vi "FromRepo.vi"(8 "error in":errorcluster, 9 "from repo cluster":T2, 10 "repository in":refnum<class "NISE_CEF_Repository.lvclass">, 11 "node in":refnum<class "VI modification collection.lvclass">) -> (0 "error out":errorcluster, 2 "repository out":refnum<class "NISE_CEF_Repository.lvclass">, 3 "node":T1)   [LabVIEW 2013, in "VI modification collection.lvclass"]
doc: "Grabs information from the Repo and stores it in the nodes."
uses:
  VI modification collection.lvclass
  <vilib>/CEF_TreeControl/Repository/NISE_CEF_Repository.lvclass
  <vilib>/CEF_TreeControl/Node/FromRepoCluster.ctl
  <vilib>/CEF_TreeControl/Node/NodeRef.ctl
  <vilib>/CEF_TreeControl/Node/NISE_CEF_Node.lvclass
  Modifier UI/modification container/modification container.lvclass
  Modifier UI/modification container/modification container.lvclass/modification container.ctl
  VI modification.lvclass
  Modifier UI/modification container/Read mods.vi
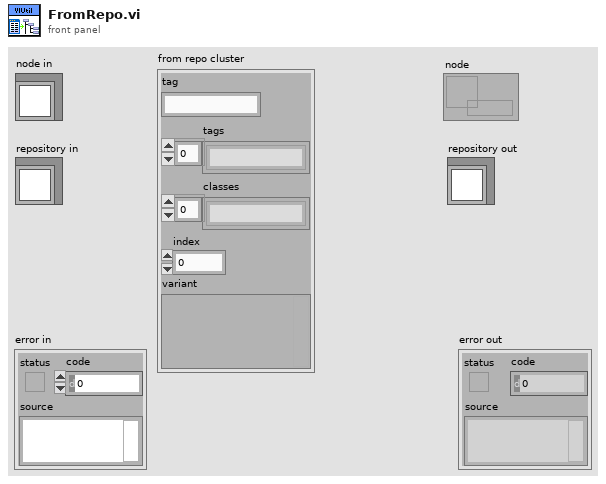
[diagram p1: front panel]
types:
  T1 = typedef "NISE_CEF_Node.lvclass/NodeRef.ctl" = refnum<data-value>
  T2 = typedef "NISE_CEF_Node.lvclass/FromRepoCluster.ctl" = cluster{"tag":string, "tags":string[], "classes":string[], "index":i32, "variant":variant}
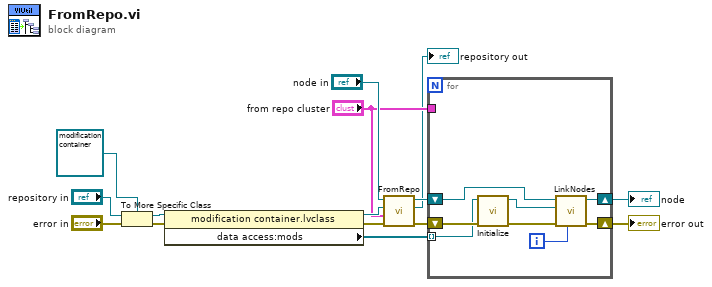
[diagram p0: block diagram]
diagram:
  n1 = To More Specific Class(target class=refnum<class "modification container.lvclass"> refnum ("modification container.lvclass"), reference="repository in", error in="error in") -> (specific class reference=w9:refnum<class "modification container.lvclass">, error out=w11:errorcluster)
  n2 = property class="modification container.lvclass"(reference=w9, error in=w11) -> (reference out=w12:refnum<class "modification container.lvclass">, error out=w13:errorcluster, "data access:mods"=w3:refnum<class "VI modification.lvclass">[])
  n3 = call-parent "FromRepo.vi"("error in"=w13, "from repo cluster"="from repo cluster", "repository in"=w12, "node in"="node in") -> ("error out"=w5:errorcluster, "repository out"=→"repository out":refnum<class "NISE_CEF_Repository.lvclass">, "node"=w7:T1)  [unwired: 5 in]
  n4 = for {
    shift-right: [w22] -> w6
    shift-left: w7 -> [w23]
    shift-right: [w20] -> w4
    shift-left: w5 -> [w19]
    tunnel: w3 -> [w18] mode=indexing
    tunnel: "from repo cluster" -> [_]
    i -> [w21]
    n5 = call-dynamic "Initialize.vi"("error in"=w19, "node in"=w18) -> ("error out"=w16:errorcluster, "data value reference"=w17:T1)  [unwired: 7 in, 1 out]
    n6 = call <vilib>:"LinkNodes.vi"("index"=w21, "error in"=w16, "child in"=w17, "parent in"=w23) -> ("error out"=w20:errorcluster, "parent out"=w22:T1)  [unwired: 5 in, 1 out]
  }
  "error out" <- w4
  "node" <- w6
